vi "plot_lifetime.vi"(7 "Spinal Column Out":T1={"Red MOT 88 Inputs"={"Active Device"="", "Active Channels"=[], "Waveform Parameters"=[], "Active Phases"=[], "Phase Times"=[], "Trigger Channel"=""}, "6713 Blue MOT"={"Active Device"="", "Active Channels"=[], "Waveform Parameters"=[], "Active Phases"=[], "Phase Times"=[], "Trigger Channel"="", "FIFO Buffer Size"=0.0}, "Instructions"=[], "Red MOT 87 Inputs"={"Active Device"="", "Active Channels"=[], "Waveform Parameters"=[], "Active Phases"=[], "Phase Times"=[], "Trigger Channel"=""}, "ODT Params"={"Waveform Parameters"=[], "Active Phases"=[], "Active Channels"=[], "Phase Times (s)"=[], "Active Device"="", "Trigger Channel"="", "Evaporation Phase"=0.0, "Evaporation Channel"=0.0}, "Agilent E3631A Settings"={"VISA resource name"="", "Voltage Set (6V max)"=0.0, "Current Set (5A max)"=0.0, "Voltage Set (25V max)"=0.0, "Current Set (1A max)"=0.0}, "PixelFly Initialization"={"Exposure mode"=0, "exp time"=0, "exp level"=0, "gain"=0, "boardid in"=0, "offset"=0, "V bin"=0, "H bin"=0, "trigger"=FALSE, "Bit depth"=0}, "Scan Parameters"={"Initial Values"=[], "Final Values"=[], "Step Sizes"=[], "Parameters to Change"=[], "Channels to Change"=[], "Number of Parameters to Scan"=0, "Parameter Nickname (no spaces)"=[], "Scan Base Name"="", "Raw_Data Folder"=path "", "ROI Parameters"={"Background Radius"=0.0, "Atom Radius"=0.0, "X Center"=0.0, "Y Center"=0.0}, "Drop Time (ms)"=0.0, "ODT VCA 1 Channel"=0.0, "ODT VCA 2 Channel"=0.0, "Phases To Change"=[], "Scan Pulseblaster Channel With Parameter"={"Change PB Time Toggle"=FALSE, "PB Channel"=0.0, "Parameter Number"=0.0}, "Preserve Waveform\nContinuity"=FALSE, "Generated Array Type"=enum."Custom Array From File", "Principle Quantum #"=0, "Angular Momentum"=enum."s", "Ramp Delay Channel"=0, "ODT Hold Channel"=0, "MCS ROI Min"=0, "MCS ROI Max"=0, "Master Batch Fourth Column"=0.0}, "MCS Parameters"={"Scan Length (Bins)"=0.0, "Dwell Time (s)"=0.0, "Gate Channel Settings"={"Threshold (V)"=0.0, "Edge"=enum."Falling", "Input Impedence"=enum."1k Ohm"}, "Trig Channel Settings"={"Threshold (V)"=0.0, "Edge"=enum."Falling", "Input Impedence"=enum."1k Ohm"}, "Input 1 Settings"={"Threshold (V)"=0.0, "Edge"=enum."Falling", "Input Impedence"=enum."1k Ohm"}, "Input 2 Settings"={"Threshold (V)"=0.0, "Edge"=enum."Falling", "Input Impedence"=enum."1k Ohm"}, "Number of Sweeps"=0, "Number of Sequential Cycles"=0.0, "Number of Sequences"=0.0, "Sweep Preset"=FALSE, "Sequential Mode"=FALSE, "DAC 1 Ramp Settings"={"Ramp Mode"=enum."Fixed", "Ramp Start Value (V)"=0.0, "Ramp Length (Steps)"=0, "Step Width (bins)"=0, "Step Size (V)"=0.0}, "DAC 2 Output (V)"=0.0, "SYNC Output"=enum."40 MHz Clock", "ROI Min"=0, "ROI Max"=0, "Dual MCS Mode"=FALSE, "DAC 2 Toggle"=FALSE, "MCS on/off"=FALSE, "ROI Max 2"=1, "ROI Min 2"=0, "Sum ROI Only"=FALSE, "Use ROI For \nEach Loop"=FALSE}, "PicoScope"={"Channel A Settings"={"Enabled"=FALSE, "Coupling"=0, "Range"=0, "Analogue Offset"=0.0}, "Channel B Settings"={"Enabled"=FALSE, "Coupling"=0, "Range"=0, "Analogue Offset"=0.0}, "Trigger Options"={"Trigger Enabled"=FALSE, "Trigger Source"=enum."Channel A", "Trigger Threshold (-5 to 5 V)"=0.0, "Trigger Slope"=0, "Trigger Delay (ms)"=0.0, "Auto Trigger Time (ms)"=0}, "Pico Scope Inititalization Settings"={"USB Power"=FALSE, "Use Serial Number"=FALSE, "Resolution"=0, "Serial Number"="", "Handle"=0}, "Use PicoScope?"=FALSE, "Acquisition Settings"={"Pre Trigger Time (s)"=0.0, "Post Trigger Time (s)"=0.0, "Resolution (s)"=0.0, "Four Channel Device"=FALSE, "Number of Captures"=0.0}}, "Ramp Delay Settings"={"Insert Delays"=FALSE, "Number of loops"=0, "Insert after instruction"=0, "Random"=FALSE, "Initial Delay Time (s)"=0.0, "Final Delay Time (s)"=0.0, "Delay Step (s)"=0.0, "Delay Column"=0.0, "Loop Hold Column"=0.0, "Field Ramp Column"=0.0, "Excitation Column"=0.0, "Hold + Delay + Excitation Time"=0.0, "Ascending/Descending"=FALSE, "Subroutine A"=[]}, "6229 Green Lattice Inputs"={"Active Device"="", "Active Channels"=[], "Waveform Parameters"=[], "Active Phases"=[], "Phase Times"=[], "Trigger Channel"="", "FIFO Buffer Size"=0.0}, "Synth Controls 1"={"Channel Settings"=[], "Active Channels"=[], "COM Port"="", "Table Mode"={"Table Mode On/Off"=FALSE, "Initial Frequency (MHz)"=0.0, "FinalFreq"=0.0, "Frequency Step (MHz)"=0.0, "Ascending/Descending"=FALSE, "Random"=FALSE}}, "Synth Controls 2"={"Channel Settings"=[], "Active Channels"=[], "COM Port"="", "Table Mode"={"Table Mode On/Off"=FALSE, "Initial Frequency (MHz)"=0.0, "FinalFreq"=0.0, "Frequency Step (MHz)"=0.0, "Ascending/Descending"=FALSE, "Random"=FALSE}}, "Indicator References"={"Blue MOT Waveform Graph"=refnum, "Red 88 Waveform Graph"=refnum, "Red 87 Waveform Graph"=refnum, "ODT Waveform Graph"=refnum, "Green Lattice Waveform Graph"=refnum, "Agilent E3631A Measurements"=refnum}} {"Red MOT 88 Inputs"."Phase Times" format="%.0p"; "Red MOT 88 Inputs"."Waveform Parameters"."Degree" min=1; "6713 Blue MOT"."Phase Times" format="%.3f"; "Instructions"."Time (s)" min=5e-08 format="%.2p"; "Instructions"."Op Code" items=["Continue", "Stop", "Loop", "End Loop", "JSR", "RTS", "Go To", "Long Delay", "Wait"]; "Instructions"."Instruct Data" format="%#.2p"; "Red MOT 87 Inputs"."Phase Times" format="%.0p"; "Red MOT 87 Inputs"."Waveform Parameters"."Degree" min=1; "ODT Params"."Evaporation Channel" min=0.0 max=1.0 step=1.0; "ODT Params"."Evaporation Phase" min=0.0 max=4.0 step=1.0; "ODT Params"."Phase Times (s)" format="%#_6p"; "Agilent E3631A Settings"."Current Set (1A max)" format="%.3g"; "Agilent E3631A Settings"."Voltage Set (25V max)" format="%.3g"; "Agilent E3631A Settings"."Current Set (5A max)" format="%.3g"; "Agilent E3631A Settings"."Voltage Set (6V max)" format="%.3g"; "PixelFly Initialization"."Bit depth" items=["2"=1]; "PixelFly Initialization"."H bin" items=["1", "2"]; "PixelFly Initialization"."V bin" items=["1", "2"]; "PixelFly Initialization"."boardid in" min=0 max=3 step=1; "PixelFly Initialization"."gain" items=["Low (X1)", "High (X2)"]; "PixelFly Initialization"."exp level" min=0 max=255 step=1; "PixelFly Initialization"."exp time" min=1 max=10000; "PixelFly Initialization"."Exposure mode" items=["Asynch shutter", "Double shot", "Video mode", "Auto exposure"]; "Scan Parameters"."Drop Time (ms)" min=1.0; "Scan Parameters"."Number of Parameters to Scan" min=1; "MCS Parameters"."ROI Max 2" min=1; "MCS Parameters"."ROI Min 2" min=0; "MCS Parameters"."ROI Max" min=1; "MCS Parameters"."ROI Min" min=0; "MCS Parameters"."DAC 2 Output (V)" min=-10.0 max=10.0 step=0.00488; "MCS Parameters"."DAC 1 Ramp Settings"."Step Size (V)" min=0.0 max=10.0 step=0.00244 format="%#_4g"; "MCS Parameters"."DAC 1 Ramp Settings"."Step Width (bins)" min=1; "MCS Parameters"."DAC 1 Ramp Settings"."Ramp Length (Steps)" min=1; "MCS Parameters"."DAC 1 Ramp Settings"."Ramp Start Value (V)" min=0.0 max=10.0 step=0.00244; "MCS Parameters"."Number of Sweeps" min=0 format="%.0p"; "MCS Parameters"."Input 2 Settings"."Threshold (V)" min=-2.5 max=2.5 step=0.001; "MCS Parameters"."Input 1 Settings"."Threshold (V)" min=-2.5 max=2.5 step=0.001; "MCS Parameters"."Trig Channel Settings"."Threshold (V)" min=-2.5 max=2.5 step=0.001; "MCS Parameters"."Gate Channel Settings"."Threshold (V)" min=-2.5 max=2.5 step=0.001; "MCS Parameters"."Dwell Time (s)" min=1e-07 step=2.5e-08 format="%#_6p"; "MCS Parameters"."Scan Length (Bins)" min=64.0 max=524288.0 format="%#_7f"; "PicoScope"."Acquisition Settings"."Resolution (s)" min=8e-09 max=34.36 step=8e-09 format="%#_6p"; "PicoScope"."Acquisition Settings"."Post Trigger Time (s)" min=0.0 format="%#_6p"; "PicoScope"."Acquisition Settings"."Pre Trigger Time (s)" min=0.0 format="%#_6p"; "PicoScope"."Pico Scope Inititalization Settings"."Resolution" items=["8-bit", "12-bit", "14-bit", "15-bit (max. 2 ch.)", "16-bit (max. 1 ch.)"]; "PicoScope"."Trigger Options"."Trigger Slope" items=["Rising"=2, "Falling"=3]; "PicoScope"."Channel B Settings"."Range" items=["10 mV", "20 mV", "50 mV", "100 mV", "200 mV", "500 mV", "1 V", "2 V", "5 V", "10 V", "20 V", "50 V ", "100 V"]; "PicoScope"."Channel B Settings"."Coupling" items=["AC", "DC"]; "PicoScope"."Channel A Settings"."Range" items=["10 mV", "20 mV", "50 mV", "100 mV", "200 mV", "500 mV", "1 V", "2 V", "5 V", "10 V", "20 V", "50 V ", "100 V"]; "PicoScope"."Channel A Settings"."Coupling" items=["AC", "DC"]; "Ramp Delay Settings"."Subroutine A"."Time (s)" min=5e-08 format="%.2p"; "Ramp Delay Settings"."Subroutine A"."Op Code" items=["Continue", "Stop", "Loop", "End Loop", "JSR", "RTS", "Go To", "Long Delay", "Wait"]; "Ramp Delay Settings"."Subroutine A"."Instruct Data" format="%#.2p"; "Ramp Delay Settings"."Insert after instruction" min=0; "Ramp Delay Settings"."Delay Step (s)" min=5e-08 format="%#_6p"; "Ramp Delay Settings"."Final Delay Time (s)" min=5e-08 format="%#_6p"; "Ramp Delay Settings"."Initial Delay Time (s)" min=5e-08 format="%#_6p"; "6229 Green Lattice Inputs"."Phase Times" format="%.3f"; "6229 Green Lattice Inputs"."Waveform Parameters"."Degree" min=1}, 10 "Tau Array":dbl[](array[numeric]), 11 "MCS Counts Out":u32[][](graph)=[[0, 0, 0, 0, 0, 0, 0, 0, 0, 0, 0, 0, 0, 0, 0, 0, 0, 0, 0, 0, 0, 0, 0, 0, 0, 0, 0, 0, 0, 0, 0, 0, 0, 0, 0, 0, 0, 0, 0, 0, 0, 0, 0, 0, 0, 0, 0, 0, 0, 0, 0, 0, 0, 0, 0, 0, 0, 0, 0, 0, 0, 0, 0, 0, 0, 0, 0, 0, 0, 0, 0, 0, 0, 1, 1, 0, 0, 0, 0, 0, 2, 0, 0, 0, 0, 0, 0, 0, 0, 0, 0, 0, 0, 1, 3, 1, 0, 0, 0, 0, 0, 0, 0, 0, 0, 0, 0, 0, 0, 0, 0, 0, 0, 0, 0, 0, 0, 0, 0, 0, 0, 0, 0, 0, 0, 0, 0, 0, 0, 0, 0, 0, 0, 0, 0, 0, 0, 0, 0, 0, 0, 0, 0, 0, 0, 0, 0, 0, 0, 0, 0, 0, 0, 0, 0, 0, 0, 0, 0, 0, 0, 0, 0, 0, 0, 0, 0, 0, 0, 0, 0, 0, 0, 0, 1, 0, 0, 0, 0, 0, 0, 0, 0, 0, 0, 0, 0, 0, 0, 0, 0, 0, 0, 0, 0, 0, 0, 0, 0, 0, 0, 0, 0, 0, 0, 0, 0, 0, 0, 0, 0, 0, 0, 0, 0, 0, 0, 0, 0, 0, 0, 0, 0, 0, 0, 0, 0, 0, 0, 0, 0, 0, 0, 0, 0, 0, 0, 0, 0, 0, 0, 0, 0, 0, 0, 0, 0, 0, 0, 0]]) -> (2 "Array":u32[][](array[numeric]), 3 "XY Graph":cluster{"Tau Array":dbl[], u32[]}[](graph))   [LabVIEW 2015]
uses:
  Controls/Spinal Column/spinal_column.ctl
  6733_Red_MOT/6733_control_panel.ctl
  6733_Red_MOT/6733_waveform_parameter_array.ctl
  6733_Red_MOT/6733_waveform_item.ctl
  6733_Red_MOT/Neutral_voltage_conversion_control.ctl
  Controls/6713/6713_waveform_generation.ctl
  Controls/6713/6713_waveform_parameter_array.ctl
  Controls/6713/6713_static_waveform_item.ctl
  Controls/PulseBlaster/Instructions_Cluster.ctl
  Neutral_DAQ/6221 arb waveforms/6221_panel.ctl
  Neutral_DAQ/6221 arb waveforms/6221_waveform_param.ctl
  Controls/Agilent E3631A/Settings_Control.ctl
  Controls/PixelFly/Camera_Initialization.ctl
  Controls/ScanParameters/ScanParametersPanel.ctl
  Controls/ScanParameters/ParameterToChange.ctl
  Controls/ScanParameters/ROI_set.ctl
  Controls/ScanParameters/ScanPBandParam.ctl
  Controls/MCS/mcs_control_panel.ctl
  Controls/MCS/mcs_channel.ctl
  Controls/MCS/ramp_control.ctl
  Controls/PicoScope/pico_control_panel.ctl
  Controls/PicoScope/pico_channel_settings.ctl
  Controls/PicoScope/pico_trigger.ctl
  Controls/PicoScope/pico_init_settings.ctl
  Controls/PulseBlaster/delay_control_3..ctl
  Controls/6229/6229_arb_waveform_generation.ctl
  Controls/Synth_409b/Synth_controls.ctl
  Controls/Synth_409b/synth_channel.ctl
  Controls/Synth_409b/table_mode.ctl
panel:
  # "Channel 0"
  # "Channel 1"
  # "Channel 2"
  # "Channel 3"
  # "Channel 4"
  # "Channel 5"
  # "Channel 7"
  # "Channel 7"
  # "(0) 689 Center Freq"
  # "(1) 689 Dither Amp"
  # "(2) 689 Power Lock"
  # "(3) Red MOT Field Grad"
  # "Channel 0"
  # "Channel 1"
  # "Channel 2"
  # "Channel 3"
  # "Channel 4"
  # "Channel 5"
  # "Channel 7"
  # "Channel 7"
  # "6V Output Settings"
  # "25V Output Settings"
  # "Select a PB Channel to set with a phase time\nfor evaporation or whatever"
  # "(0) Arm A"
  # "(1) Arm B"
  # "(2) Arm C"
  # "(3) Unused"
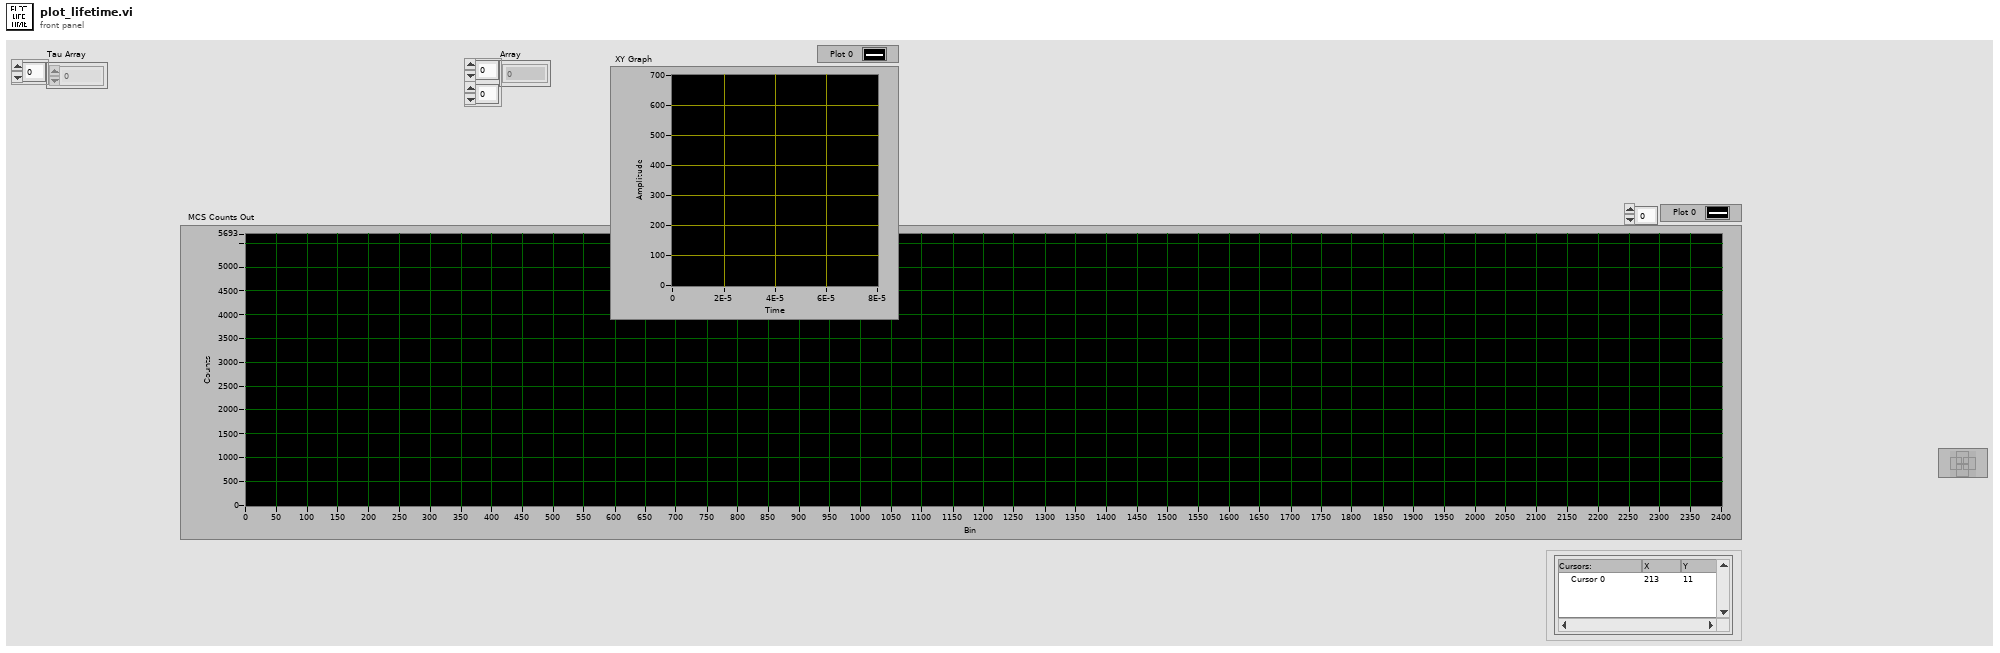
[diagram p1: front panel]
types:
  T1 = typedef "spinal_column.ctl" = cluster{"Red MOT 88 Inputs":T2, "6713 Blue MOT":T6, "Instructions":T9, "Red MOT 87 Inputs":T2, "ODT Params":T10, "Agilent E3631A Settings":T12, "PixelFly Initialization":T13, "Scan Parameters":T14, "MCS Parameters":T18, "PicoScope":T21, "Ramp Delay Settings":T25, "6229 Green Lattice Inputs":T26, "Synth Controls 1":T27, "Synth Controls 2":T27, "Indicator References":cluster{"Blue MOT Waveform Graph":refnum<vi>, "Red 88 Waveform Graph":refnum<vi>, "Red 87 Waveform Graph":refnum<vi>, "ODT Waveform Graph":refnum<vi>, "Green Lattice Waveform Graph":refnum<vi>, "Agilent E3631A Measurements":refnum<vi>}}
  T2 = typedef "6733_control_panel.ctl" = cluster{"Active Device":string, "Active Channels":bool[], "Waveform Parameters":T3, "Active Phases":bool[], "Phase Times":dbl[], "Trigger Channel":tag}
  T3 = typedef "6733_waveform_parameter_array.ctl" = T4[][]
  T4 = typedef "6733_waveform_item.ctl" = cluster{"Function":enum16{"Polynomial", "Exponential", "Constant"}, "Initial":dbl, "Final":dbl, "Degree":i8, "Nickname":string, "Conversion":T5, "Constant":dbl}
  T5 = typedef "Neutral_voltage_conversion_control.ctl" = enum16{"Volts", "B Field Grad (G/cm)", "Red MOT Center Freq (MHz)", "Red Dither Pk(kHz)", "Red Power (mW)", "ODT Sheet Trap Power (W)", "ODT Loading Trap Power (W)"}
  T6 = typedef "6713_waveform_generation.ctl" = cluster{"Active Device":string, "Active Channels":bool[], "Waveform Parameters":T7, "Active Phases":bool[], "Phase Times":dbl[], "Trigger Channel":tag, "FIFO Buffer Size":dbl}
  T7 = typedef "6713_waveform_parameter_array.ctl" = T8[][]
  T8 = typedef "6713_static_waveform_item.ctl" = cluster{"Constant":dbl, "Nickname":string, "Conversion":T5}
  T9 = typedef "Instructions_Cluster.ctl" = cluster{"Instruct Data":i32, "Op Code":i32, "Flags":bool[], "Comments":string, "Time (s)":dbl, "Column Number":string, "Array":string[]}[]
  T10 = typedef "6221_panel.ctl" = cluster{"Waveform Parameters":T11[][], "Active Phases":bool[], "Active Channels":bool[], "Phase Times (s)":dbl[], "Active Device":string, "Trigger Channel":tag, "Evaporation Phase":dbl, "Evaporation Channel":dbl}
  T11 = typedef "6221_waveform_param.ctl" = cluster{"Initial Value":dbl, "Final Value":dbl, "Tau":dbl, "Eta":dbl, "Nickname":string, "Enum":enum16{"Volts to Volts", "Power Law", "Evaporation Formula"}, "Conversion":T5}
  T12 = typedef "Settings_Control.ctl" = cluster{"VISA resource name":refnum<visa-resource-name>, "Voltage Set (6V max)":dbl, "Current Set (5A max)":dbl, "Voltage Set (25V max)":dbl, "Current Set (1A max)":dbl}
  T13 = typedef "Camera_Initialization.ctl" = cluster{"Exposure mode":u16, "exp time":i32, "exp level":i32, "gain":i32, "boardid in":i32, "offset":i32, "V bin":i32, "H bin":i32, "trigger":bool, "Bit depth":i32}
  T14 = typedef "ScanParametersPanel.ctl" = cluster{"Initial Values":dbl[], "Final Values":dbl[], "Step Sizes":dbl[], "Parameters to Change":T15[], "Channels to Change":dbl[], "Number of Parameters to Scan":i32, "Parameter Nickname (no spaces)":string[], "Scan Base Name":string, "Raw_Data Folder":path, "ROI Parameters":T16, "Drop Time (ms)":dbl, "ODT VCA 1 Channel":dbl, "ODT VCA 2 Channel":dbl, "Phases To Change":dbl[], "Scan Pulseblaster Channel With Parameter":T17, "Preserve Waveform\nContinuity":bool, "Generated Array Type":enum16{"Custom Array From File", "Default (old way)"}, "Principle Quantum #":i32, "Angular Momentum":enum16{"s", "p", "d", "f", "g", "h"}, "Ramp Delay Channel":i32, "ODT Hold Channel":i32, "MCS ROI Min":i32, "MCS ROI Max":i32, "Master Batch Fourth Column":dbl}
  T15 = typedef "ParameterToChange.ctl" = enum16{"Delay single delay time", "Dummy Variable", "Delay Exposure", "PB Loops", "Number of Delay Loops", "Subroutine A Time", "Subroutine B Time", "Synth Amplitude", "Synth Frequency", "Synth Phase", "ODT Params Phase Time", "ODT Params Tau", "ODT Params Final Voltage", "ODT Params Initial Voltage", "ODT Params Eta", "Red Mot 88 Phase Time", "Red Mot 87 Phase Time", "Red Mot 88 Final Voltage", "Red Mot 88 Initial Voltage", "Red Mot 87 Final Voltage", "Red Mot 87 Initial Voltage", "PulseBlaster", "6713 Voltage"}
  T16 = typedef "ROI_set.ctl" = cluster{"Background Radius":dbl, "Atom Radius":dbl, "X Center":dbl, "Y Center":dbl}
  T17 = typedef "ScanPBandParam.ctl" = cluster{"Change PB Time Toggle":bool, "PB Channel":dbl, "Parameter Number":dbl}
  T18 = typedef "mcs_control_panel.ctl" = cluster{"Scan Length (Bins)":dbl, "Dwell Time (s)":dbl, "Gate Channel Settings":T19, "Trig Channel Settings":T19, "Input 1 Settings":T19, "Input 2 Settings":T19, "Number of Sweeps":i32, "Number of Sequential Cycles":dbl, "Number of Sequences":dbl, "Sweep Preset":bool, "Sequential Mode":bool, "DAC 1 Ramp Settings":T20, "DAC 2 Output (V)":dbl, "SYNC Output":enum16{"40 MHz Clock", "Gate Disc Signal", "Trigger Disc Signal", "Counter 1 Disc Signal", "Counter 2 Disc Signal", "Definitely Not Used", "Not Used", "1 kHz Signal", "Also Not Used", "MCS On/Off", "End of Time Bin", "Ramp Increment Trig", "Step Count Trigger", "'GO'-Line", "Ramp Down Trigger", "Logic 1"}, "ROI Min":i32, "ROI Max":i32, "Dual MCS Mode":bool, "DAC 2 Toggle":bool, "MCS on/off":bool, "ROI Max 2":i32, "ROI Min 2":i32, "Sum ROI Only":bool, "Use ROI For \nEach Loop":bool}
  T19 = typedef "mcs_channel.ctl" = cluster{"Threshold (V)":dbl, "Edge":enum16{"Falling", "Rising"}, "Input Impedence":enum16{"1k Ohm", "50 Ohm"}}
  T20 = typedef "ramp_control.ctl" = cluster{"Ramp Mode":enum16{"Fixed", "Triangle", "Sawtooth"}, "Ramp Start Value (V)":dbl, "Ramp Length (Steps)":i32, "Step Width (bins)":i32, "Step Size (V)":dbl}
  T21 = typedef "pico_control_panel.ctl" = cluster{"Channel A Settings":T22, "Channel B Settings":T22, "Trigger Options":T23, "Pico Scope Inititalization Settings":T24, "Use PicoScope?":bool, "Acquisition Settings":cluster{"Pre Trigger Time (s)":dbl, "Post Trigger Time (s)":dbl, "Resolution (s)":dbl, "Four Channel Device":bool, "Number of Captures":dbl}}
  T22 = typedef "pico_channel_settings.ctl" = cluster{"Enabled":bool, "Coupling":i16, "Range":u16, "Analogue Offset":sgl}
  T23 = typedef "pico_trigger.ctl" = cluster{"Trigger Enabled":bool, "Trigger Source":enum16{"Channel A", "Channel B", "Channel C", "Channel D", "Ext."}, "Trigger Threshold (-5 to 5 V)":dbl, "Trigger Slope":u16, "Trigger Delay (ms)":dbl, "Auto Trigger Time (ms)":i16}
  T24 = typedef "pico_init_settings.ctl" = cluster{"USB Power":bool, "Use Serial Number":bool, "Resolution":i32, "Serial Number":string, "Handle":i16}
  T25 = typedef "delay_control_3..ctl" = cluster{"Insert Delays":bool, "Number of loops":i32, "Insert after instruction":i32, "Random":bool, "Initial Delay Time (s)":dbl, "Final Delay Time (s)":dbl, "Delay Step (s)":dbl, "Delay Column":dbl, "Loop Hold Column":dbl, "Field Ramp Column":dbl, "Excitation Column":dbl, "Hold + Delay + Excitation Time":dbl, "Ascending/Descending":bool, "Subroutine A":T9}
  T26 = typedef "6229_arb_waveform_generation.ctl" = cluster{"Active Device":string, "Active Channels":bool[], "Waveform Parameters":T3, "Active Phases":bool[], "Phase Times":dbl[], "Trigger Channel":tag, "FIFO Buffer Size":dbl}
  T27 = typedef "Synth_controls.ctl" = cluster{"Channel Settings":T28[], "Active Channels":bool[], "COM Port":refnum<visa-resource-name>, "Table Mode":T29}
  T28 = typedef "synth_channel.ctl" = cluster{"Voltage (Amp.) ":dbl, "Frequency (MHz)":dbl, "Phase (deg)":dbl, "Nickname":string}
  T29 = typedef "table_mode.ctl" = cluster{"Table Mode On/Off":bool, "Initial Frequency (MHz)":dbl, "FinalFreq":dbl, "Frequency Step (MHz)":dbl, "Ascending/Descending":bool, "Random":bool}
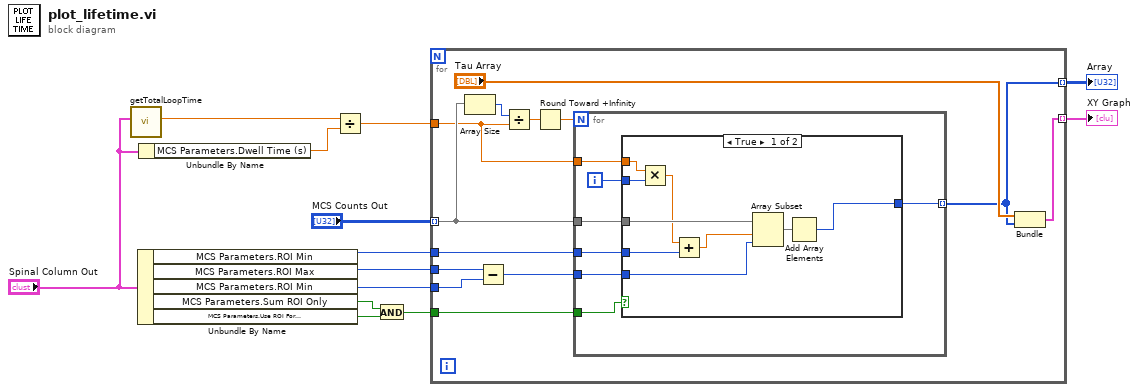
[diagram p0: block diagram]
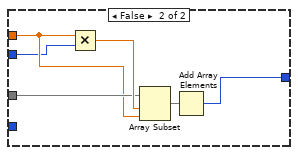
[diagram p2: hidden frame]
diagram:
  n1 = call "getTotalLoopTime.vi"("Spinal Column Out"="Spinal Column Out") -> ("Total Loop Time"=w2:dbl)  [unwired: 10 in]
  n2 = Unbundle By Name("Spinal Column Out") -> ("MCS Parameters.ROI Min"=w5:i32, "MCS Parameters.ROI Max"=w6:i32, "MCS Parameters.ROI Min"=w7:i32, "MCS Parameters.Sum ROI Only"=w10:bool, "MCS Parameters.Use ROI For \nEach Loop"=w9:bool)
  n3 = Unbundle By Name("Spinal Column Out") -> ("MCS Parameters.Dwell Time (s)"=w1:dbl)
  n4 = Divide(x=w2, y=w1) -> (x/y=w4:dbl)
  n5 = And(x=w10, y=w9) -> (x .and. y?=w8:bool)
  n6 = for {
    tunnel: "MCS Counts Out" -> [w25] mode=indexing
    tunnel: [w23] -> w12 mode=indexing
    tunnel: [w22] -> w11 mode=indexing
    tunnel: w8 -> [w21]
    tunnel: w7 -> [w20]
    tunnel: w6 -> [w19]
    tunnel: w5 -> [w18]
    tunnel: w4 -> [w14]
    n7 = Array Size(array=w25) -> (size(s)=w26:i32)
    n8 = Subtract(x=w19, y=w20) -> (x-y=w17:i32)
    n9 = Divide(x=w26, y=w14) -> (x/y=w15:dbl)
    n10 = Round Toward +Infinity(x=w15) -> (ceil(x): smallest int >= x=w16:dbl)
    n11 = for {
      N: w16 -> [_]
      tunnel: w25 -> [w33]
      tunnel: w14 -> [w32]
      tunnel: [w31] -> w23 mode=indexing
      tunnel: w21 -> [w29]
      tunnel: w18 -> [w28]
      tunnel: w17 -> [w27]
      i -> [w30]
      n12 = case shown="True" w29 {
        tunnel: w33 -> [w42 w47]
        tunnel: w32 -> [w37 w45]
        tunnel: [w40 w44] -> w31
        tunnel: w30 -> [w38 w43]
        tunnel: w28 -> [w39 _]
        tunnel: w27 -> [w34 _]
        frame True {
          n13 = Multiply(x=w37, y=w38) -> (x*y=w36:dbl)
          n14 = Add(x=w36, y=w39) -> (x+y=w35:dbl)
          n15 = Array Subset(array=w42, index=w35, length=w34) -> (w41:u32[])
          n16 = Add Array Elements(numeric array=w41) -> (sum=w40:u32)
        }
        frame False {
          n17 = Multiply(x=w45, y=w43) -> (x*y=w48:dbl)
          n18 = Array Subset(array=w47, index=w48, length=w45) -> (w46:u32[])
          n19 = Add Array Elements(numeric array=w46) -> (sum=w44:u32)
        }
      }
    }
    n20 = Bundle("Tau Array"="Tau Array", w23) -> (w22:cluster{"Tau Array":dbl[], u32[]})  [unwired: 1 in]
  }
  "Array" <- w12
  "XY Graph" <- w11
